vi "Sistema.vi"() -> ()   [LabVIEW 2017]
uses:
  <vilib>/Motion/Express/_s/nimc.ex.write.writeSetpoint.axis.vi
  <vilib>/Motion/Express/_s/nimc.fb.straightLineMove.startStraightLineMove.axis.modeAbsolute.0.vi
  <vilib>/Motion/Express/_s/nimc.ex.read.readExecutionData.axis.vi
  <vilib>/Motion/BlockNode/FB.NIMotion.xnode
panel:
  in  "Velocidad":dbl=10.0 format="%#_13g"
  out "x > y?":bool=TRUE
  out "done":bool=TRUE
  in  "Posición Inicial":cluster{"X":dbl, "Y":dbl, "Z":dbl}
  in  "Array":T1(array[cluster])=[{"Tipo Movimiento"=enum."Lineal", "X"=3.0, "Y"=0.0}, {"Tipo Movimiento"=enum."Lineal", "X"=3.0, "Y"=1.0}, {"Tipo Movimiento"=enum."Lineal", "X"=1.0, "Y"=1.0}, {"Tipo Movimiento"=enum."Lineal", "X"=1.0, "Y"=5.0}, {"Tipo Movimiento"=enum."Lineal", "X"=0.0, "Y"=5.0}, {"Tipo Movimiento"=enum."Lineal", "X"=0.0, "Y"=0.0}, {"Tipo Movimiento"=enum."Lineal", "X"=7.0, "Y"=0.0}, {"Tipo Movimiento"=enum."Lineal", "X"=7.0, "Y"=5.0}, {"Tipo Movimiento"=enum."Lineal", "X"=6.0, "Y"=5.0}, {"Tipo Movimiento"=enum."Lineal", "X"=6.0, "Y"=1.0}, {"Tipo Movimiento"=enum."Lineal", "X"=5.0, "Y"=1.0}, {"Tipo Movimiento"=enum."Lineal", "X"=5.0, "Y"=5.0}, {"Tipo Movimiento"=enum."Lineal", "X"=4.0, "Y"=5.0}, {"Tipo Movimiento"=enum."Lineal", "X"=4.0, "Y"=0.0}, {"Tipo Movimiento"=enum."Lineal", "X"=12.0, "Y"=0.0}, {"Tipo Movimiento"=enum."Lineal", "X"=12.0, "Y"=1.0}, {"Tipo Movimiento"=enum."Lineal", "X"=10.5, "Y"=1.0}, {"Tipo Movimiento"=enum."Lineal", "X"=10.5, "Y"=4.0}, {"Tipo Movimiento"=enum."Lineal", "X"=12.0, "Y"=4.0}, {"Tipo Movimiento"=enum."Lineal", "X"=12.0, "Y"=5.0}, {"Tipo Movimiento"=enum."Lineal", "X"=8.0, "Y"=5.0}, {"Tipo Movimiento"=enum."Lineal", "X"=8.0, "Y"=4.0}, {"Tipo Movimiento"=enum."Lineal", "X"=9.5, "Y"=4.0}, {"Tipo Movimiento"=enum."Lineal", "X"=9.5, "Y"=1.0}, {"Tipo Movimiento"=enum."Lineal", "X"=8.0, "Y"=1.0}, {"Tipo Movimiento"=enum."Lineal", "X"=8.0, "Y"=0.0}, {"Tipo Movimiento"=enum."Lineal", "X"=15.5, "Y"=0.0}, {"Tipo Movimiento"=enum."Lineal", "X"=16.0, "Y"=0.5}, {"Tipo Movimiento"=enum."Lineal", "X"=16.0, "Y"=2.0}, {"Tipo Movimiento"=enum."Lineal", "X"=15.5, "Y"=2.5}, {"Tipo Movimiento"=enum."Lineal", "X"=14.5, "Y"=2.5}, {"Tipo Movimiento"=enum."Lineal", "X"=14.0, "Y"=3.0}, {"Tipo Movimiento"=enum."Lineal", "X"=14.0, "Y"=3.5}, {"Tipo Movimiento"=enum."Lineal", "X"=14.5, "Y"=4.0}, {"Tipo Movimiento"=enum."Lineal", "X"=15.75, "Y"=4.0}, {"Tipo Movimiento"=enum."Lineal", "X"=16.0, "Y"=4.25}, {"Tipo Movimiento"=enum."Lineal", "X"=16.0, "Y"=4.75}, {"Tipo Movimiento"=enum."Lineal", "X"=15.75, "Y"=5.0}, {"Tipo Movimiento"=enum."Lineal", "X"=13.5, "Y"=5.0}, {"Tipo Movimiento"=enum."Lineal", "X"=13.0, "Y"=4.5}, {"Tipo Movimiento"=enum."Lineal", "X"=13.0, "Y"=2.5}, {"Tipo Movimiento"=enum."Lineal", "X"=13.5, "Y"=2.0}, {"Tipo Movimiento"=enum."Lineal", "X"=14.5, "Y"=2.0}, {"Tipo Movimiento"=enum."Lineal", "X"=15.0, "Y"=1.5}, {"Tipo Movimiento"=enum."Lineal", "X"=15.0, "Y"=1.0}, {"Tipo Movimiento"=enum."Lineal", "X"=14.5, "Y"=0.5}, {"Tipo Movimiento"=enum."Lineal", "X"=13.0, "Y"=0.5}, {"Tipo Movimiento"=enum."Lineal", "X"=13.0, "Y"=0.0}, {"Tipo Movimiento"=enum."Lineal", "X"=20.0, "Y"=0.0}, {"Tipo Movimiento"=enum."Lineal", "X"=20.0, "Y"=2.0}, {"Tipo Movimiento"=enum."Lineal", "X"=22.0, "Y"=2.0}, {"Tipo Movimiento"=enum."Lineal", "X"=22.0, "Y"=3.0}, {"Tipo Movimiento"=enum."Lineal", "X"=20.0, "Y"=3.0}, {"Tipo Movimiento"=enum."Lineal", "X"=20.0, "Y"=4.0}, {"Tipo Movimiento"=enum."Lineal", "X"=22.0, "Y"=4.0}, {"Tipo Movimiento"=enum."Lineal", "X"=22.0, "Y"=5.0}, {"Tipo Movimiento"=enum."Lineal", "X"=19.0, "Y"=5.0}, {"Tipo Movimiento"=enum."Lineal", "X"=19.0, "Y"=0.0}, {"Tipo Movimiento"=enum."Lineal", "X"=26.0, "Y"=0.0}, {"Tipo Movimiento"=enum."Lineal", "X"=26.0, "Y"=1.0}, {"Tipo Movimiento"=enum."Lineal", "X"=24.0, "Y"=1.0}, {"Tipo Movimiento"=enum."Lineal", "X"=24.0, "Y"=2.0}, {"Tipo Movimiento"=enum."Lineal", "X"=26.0, "Y"=2.0}, {"Tipo Movimiento"=enum."Lineal", "X"=26.0, "Y"=3.0}, {"Tipo Movimiento"=enum."Lineal", "X"=24.0, "Y"=3.0}, {"Tipo Movimiento"=enum."Lineal", "X"=24.0, "Y"=4.0}, {"Tipo Movimiento"=enum."Lineal", "X"=26.0, "Y"=4.0}, {"Tipo Movimiento"=enum."Lineal", "X"=26.0, "Y"=5.0}, {"Tipo Movimiento"=enum."Lineal", "X"=23.0, "Y"=5.0}, {"Tipo Movimiento"=enum."Lineal", "X"=23.0, "Y"=0.0}, {"Tipo Movimiento"=enum."Lineal", "X"=27.5, "Y"=0.0}, {"Tipo Movimiento"=enum."Lineal", "X"=27.5, "Y"=2.0}, {"Tipo Movimiento"=enum."Lineal", "X"=28.0, "Y"=2.0}, {"Tipo Movimiento"=enum."Lineal", "X"=29.0, "Y"=0.0}, {"Tipo Movimiento"=enum."Lineal", "X"=30.0, "Y"=0.0}, {"Tipo Movimiento"=enum."Lineal", "X"=30.0, "Y"=1.0}, {"Tipo Movimiento"=enum."Lineal", "X"=29.0, "Y"=2.5}]
  out "Paso":i32=69
  in  "Stop Button":bool
  out "EY":dbl(slide) scale=0.0..10.0
  out "EX":dbl(slide)=23.0 scale=0.0..10.0
  out "XY Graph":cluster{dbl[], dbl[]}(graph)={[0.0, 0.426423996, 1.426315789, 2.4263157890000002, 2.999891794, 3.0, 2.997709298, 2.215789474, 1.218080176, 1.0, 1.0, 1.0, 1.0, 1.0, 1.0, 0.45789473700000005, -0.0, -0.0, -0.0, -0.0, -0.0, -0.0, -0.0, 0.005048895, 0.32563547000000004, 1.194736842, 2.194736842, 2.894736842, 3.894736842, 4.894736842, 5.894736842, 6.727090094, 6.998255176, 7.0, 7.0, 7.0, 7.0, 7.0, 7.0, 7.0, 6.557894737, 6.0, 6.0, 6.0, 6.0, 6.0, 6.0, 5.557894737, 5.0, 5.0, 5.0, 5.0, 5.0, 5.0, 5.0, 4.157894737, 4.0, 4.0, 4.0, 4.0, 4.0, 4.0, 4.0, 4.048989208, 4.516094471, 5.436842105, 6.436842105, 7.436842105, 8.436842105, 9.436842105, 10.436842105, 11.387852897, 11.920747634, 12.0, 12.0, 11.916385042, 10.936842105, 10.5, 10.5, 10.5, 10.5, 10.5, 11.063157895, 11.979542936, 12.0, 12.0, 11.995418596, 11.529091619999999, 10.531578947, 9.531578947, 8.532151623, 8.002487327, 8.0, 8.0, 8.763157895, 9.5, 9.5, 9.5, 9.5, 9.5, 9.136842105, 8.066802093, 8.0, 8.0, 8.055501693, 8.564273623, 9.515789474, 10.515789474, 11.515789474, 12.515789474, 13.515789474, 14.514486319, 15.27534626, 15.499221793, 15.990506967, 16.0, 16.0, 15.584, 15.057894737, 14.5, 14.0, 14.116, 14.607617729, 15.601898554, 15.999811191, 16.0, 15.75, 15.105263158, 14.105263158, 13.5, 13.0, 13.0, 13.0, 13.0, 13.509032779, 14.486361958, 14.990506967, 15.0, 14.5, 13.836842105, 13.001629181, 13.0, 13.092082839, 13.707674496, 14.694736842, 15.694736842, 16.694736842, 17.694736842, 18.694736842, 19.602654003, 19.987062346000002, 20.0, 20.0, 20.0, 20.111486611, 21.084210526, 21.972723915, 22.0, 22.0, 21.415789474, 20.415789474, 20.0, 20.0, 20.111486611, 21.084210526, 21.972723915, 22.0, 22.0, 21.573576004, 20.573684211, 19.573684211, 19.0, 19.0, 19.0, 19.0, 19.0, 19.0, 19.0, 19.0, 19.167646748, 19.896481666, 20.894736842, 21.894736842, 22.894736842, 23.894736842, 24.994549846, 25.780379567, 25.999747518, 26.0, 26.0, 25.315789474, 24.218080176, 24.0, 24.0, 24.284282664, 25.284210526, 25.999927862, 26.0, 25.997709298, 25.215789474, 24.218080176, 24.0, 24.0, 24.284282664, 25.284210526, 25.999927862, 26.0, 25.99898191, 25.373684211, 24.373684211, 23.3747023, 23.0, 23.0, 23.0, 23.0, 23.0, 23.0, 23.0], [0.0, 0.0, 0.0, 0.0, 0.0, 0.5421052630000001, 1.0, 1.0, 1.0, 1.004581404, 1.568565328, 2.568421053, 3.568421053, 4.563839648, 4.999855725, 5.0, 5.0, 4.721283472, 3.789473684, 2.789473684, 1.6894736840000002, 0.689840197, 0.039900739000000005, 0.0, 0.0, 0.0, 0.0, 0.0, 0.0, 0.0, 0.0, 0.0, 0.0, 0.045163897, 0.71070666, 1.7105263160000002, 2.710526316, 3.610526316, 4.587072946, 4.997899781, 5.0, 5.0, 4.621142376, 3.631578947, 2.631578947, 1.532151623, 1.002487327, 1.0, 1.0, 1.3788576240000001, 2.268421053, 2.968421053, 3.868421053, 4.801204409, 5.0, 5.0, 4.97654663, 4.28929334, 3.289473684, 2.289473684, 1.289473684, 0.334637581, 0.000180344, 0.0, 0.0, 0.0, 0.0, 0.0, 0.0, 0.0, 0.0, 0.0, 0.0, 0.0, 0.742105263, 1.0, 1.0, 1.0, 1.5263157889999999, 2.526315789, 3.526315789, 4.0, 4.0, 4.0, 4.442105263, 5.0, 5.0, 5.0, 5.0, 5.0, 5.0, 5.0, 4.557894737, 4.0, 4.0, 4.0, 3.670425848, 2.6736842110000003, 1.673684211, 1.003258362, 1.0, 1.0, 0.657894737, -0.0, -0.0, -0.0, -0.0, -0.0, -0.0, -0.0, -0.0, -0.0, -0.0, -0.0, 0.490506967, 0.963157895, 1.933197907, 2.416, 2.5, 2.5, 3.025493033, 3.616, 4.0, 4.0, 4.249811191, 4.75, 5.0, 5.0, 5.0, 5.0, 4.5, 3.9157894740000003, 2.9157894740000003, 2.5, 2.0, 2.0, 1.509493033, 1.0, 0.5, 0.5, 0.5, 0.0, 0.0, 0.0, 0.0, 0.0, 0.0, 0.0, 0.0, 0.0, 0.0, 0.05435941800000001, 0.984210526, 1.929851108, 2.0, 2.0, 2.0, 2.342105263, 3.0, 3.0, 3.0, 3.0, 3.842105263, 4.0, 4.0, 4.0, 4.342105263, 5.0, 5.0, 5.0, 5.0, 5.0, 4.839704524, 3.989473684, 2.989473684, 1.989473684, 0.989473684, 0.14976916, -0.0, -0.0, -0.0, -0.0, -0.0, -0.0, -0.0, -0.0, -0.0, -0.0, 0.442105263, 1.0, 1.0, 1.0, 1.055743306, 1.986361958, 2.0, 2.0, 2.0, 2.542105263, 3.0, 3.0, 3.0, 3.055743306, 3.986361958, 4.0, 4.0, 4.0, 4.542105263, 5.0, 5.0, 5.0, 5.0, 5.0, 4.721283472, 3.789473684, 2.789473684, 1.789473684, 0.7894736840000001, 0.068190212]}
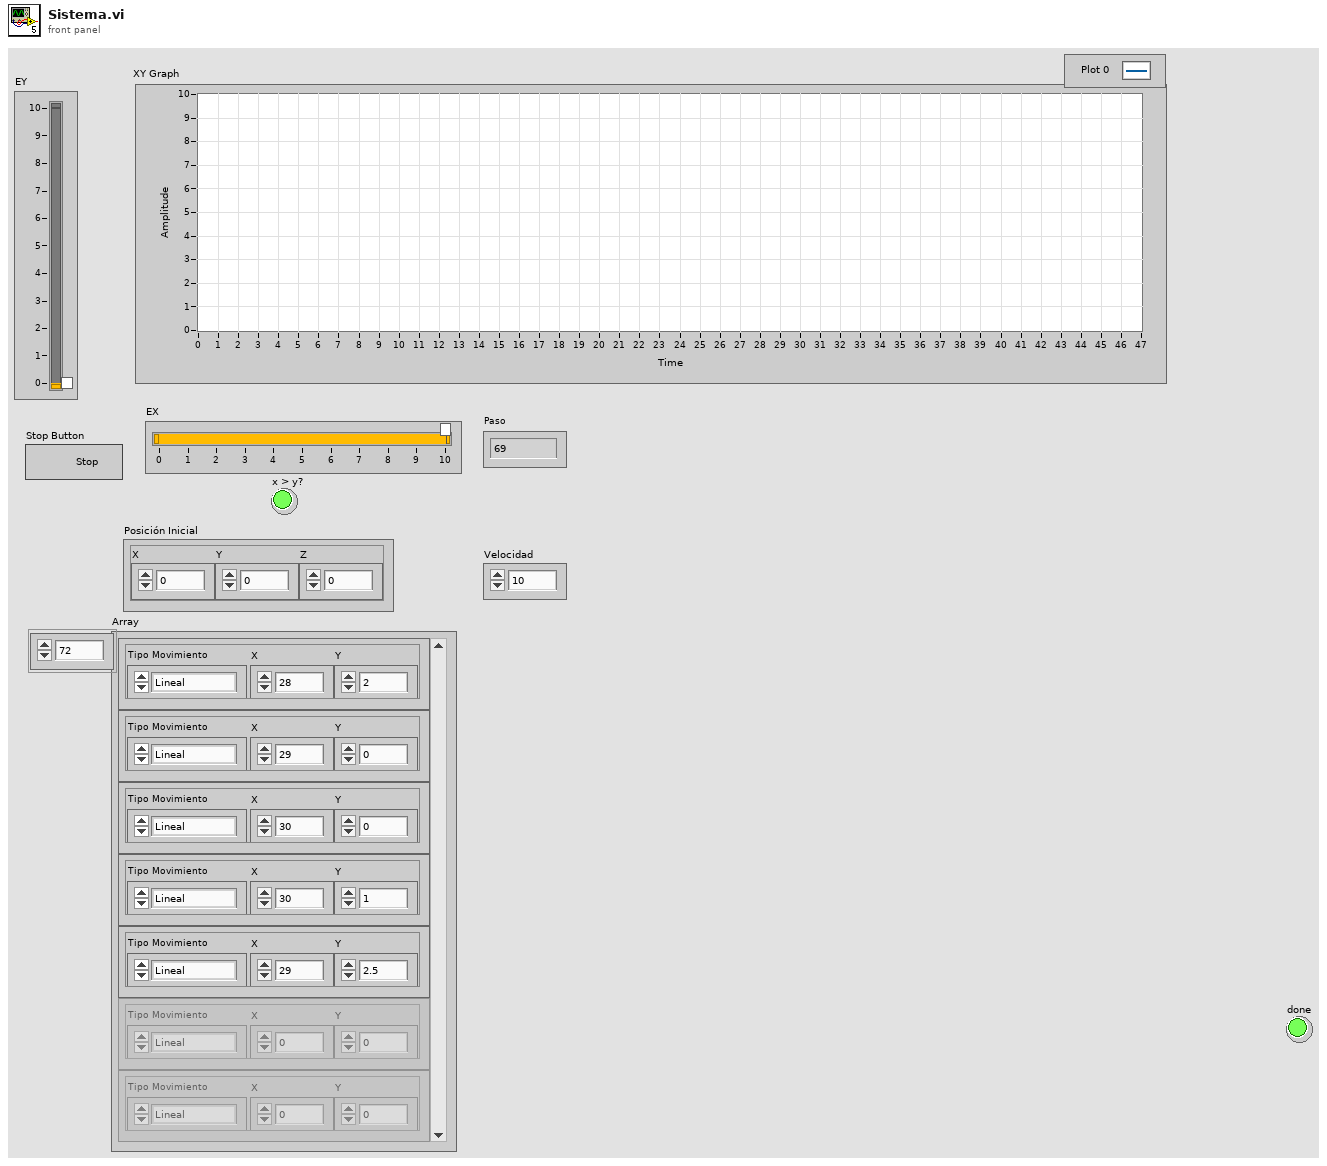
[diagram p1: front panel]
types:
  T1 = cluster{"Tipo Movimiento":enum16{"Lineal", "Circular"}, "X":dbl, "Y":dbl}[]
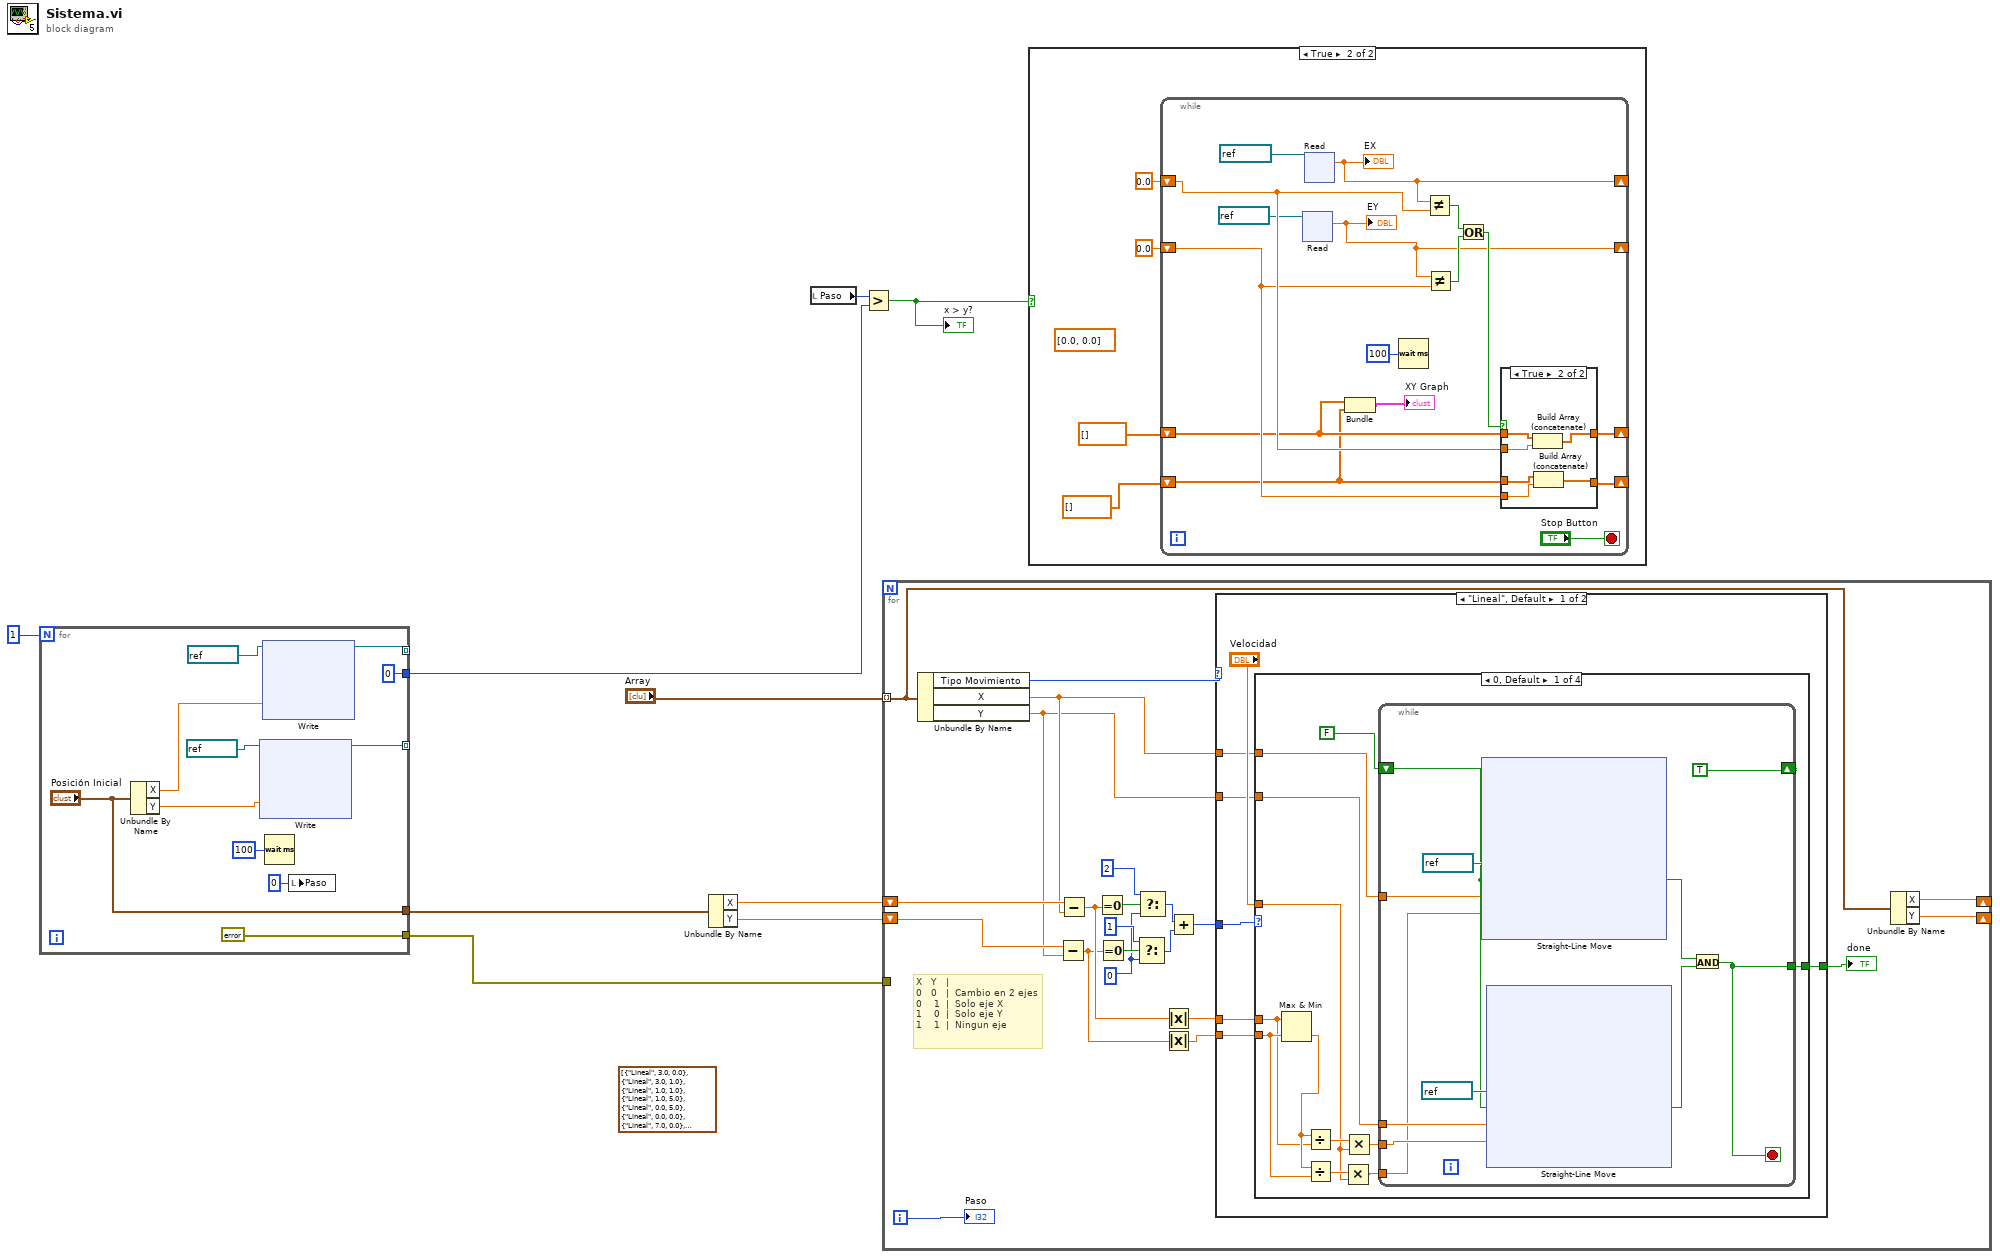
[diagram p0: block diagram]
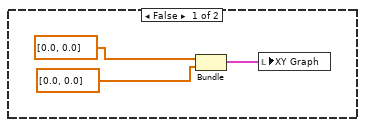
[diagram p2: hidden frame]
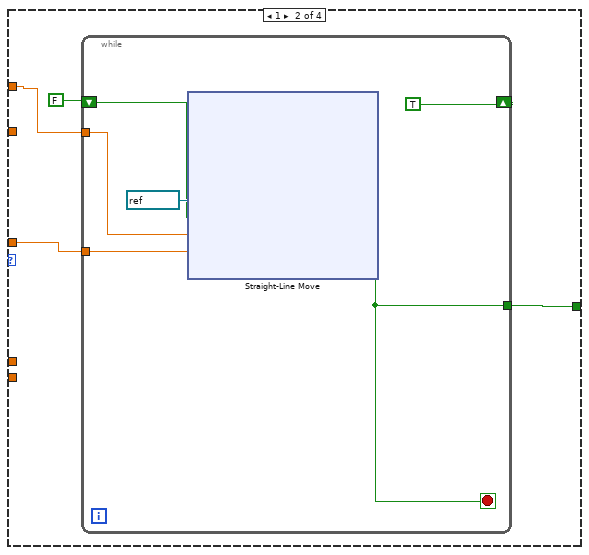
[diagram p4: hidden frame]
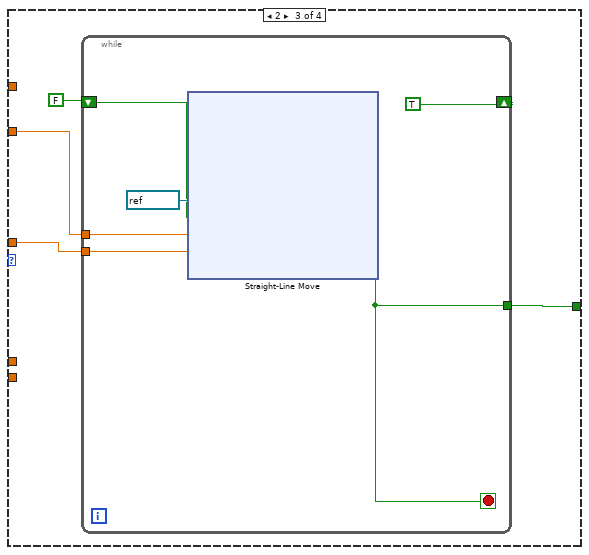
[diagram p5: hidden frame]
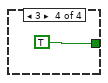
[diagram p6: hidden frame]
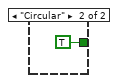
[diagram p7: hidden frame]
diagram:
  (unwired) T1 [{"Tipo Movimiento"=enum."Lineal", "X"=3.0, "Y"=0.0}, {"Tipo Movimiento"=enum."Lineal", "X"=3.0, "Y"=1.0}, {"Tipo Movimiento"=enum."Lineal", "X"=1.0, "Y"=1.0}, {"Tipo Movimiento"=enum."Lineal", "X"=1.0, "Y"=5.0}, {"Tipo Movimiento"=enum."Lineal", "X"=0.0, "Y"=5.0}, {"Tipo Movimiento"=enum."Lineal", "X"=0.0, "Y"=0.0}, {"Tipo Movimiento"=enum."Lineal", "X"=7.0, "Y"=0.0}, {"Tipo Movimiento"=enum."Lineal", "X"=7.0, "Y"=5.0}, {"Tipo Movimiento"=enum."Lineal", "X"=6.0, "Y"=5.0}, {"Tipo Movimiento"=enum."Lineal", "X"=6.0, "Y"=1.0}, {"Tipo Movimiento"=enum."Lineal", "X"=5.0, "Y"=1.0}, {"Tipo Movimiento"=enum."Lineal", "X"=5.0, "Y"=5.0}, {"Tipo Movimiento"=enum."Lineal", "X"=4.0, "Y"=5.0}, {"Tipo Movimiento"=enum."Lineal", "X"=4.0, "Y"=0.0}, {"Tipo Movimiento"=enum."Lineal", "X"=12.0, "Y"=0.0}, {"Tipo Movimiento"=enum."Lineal", "X"=12.0, "Y"=1.0}, {"Tipo Movimiento"=enum."Lineal", "X"=10.5, "Y"=1.0}, {"Tipo Movimiento"=enum."Lineal", "X"=10.5, "Y"=4.0}, {"Tipo Movimiento"=enum."Lineal", "X"=12.0, "Y"=4.0}, {"Tipo Movimiento"=enum."Lineal", "X"=12.0, "Y"=5.0}, {"Tipo Movimiento"=enum."Lineal", "X"=8.0, "Y"=5.0}, {"Tipo Movimiento"=enum."Lineal", "X"=8.0, "Y"=4.0}, {"Tipo Movimiento"=enum."Lineal", "X"=9.5, "Y"=4.0}, {"Tipo Movimiento"=enum."Lineal", "X"=9.5, "Y"=1.0}, {"Tipo Movimiento"=enum."Lineal", "X"=8.0, "Y"=1.0}, {"Tipo Movimiento"=enum."Lineal", "X"=8.0, "Y"=0.0}, {"Tipo Movimiento"=enum."Lineal", "X"=15.5, "Y"=0.0}, {"Tipo Movimiento"=enum."Lineal", "X"=16.0, "Y"=0.5}, {"Tipo Movimiento"=enum."Lineal", "X"=16.0, "Y"=2.0}, {"Tipo Movimiento"=enum."Lineal", "X"=15.5, "Y"=2.5}, {"Tipo Movimiento"=enum."Lineal", "X"=14.5, "Y"=2.5}, {"Tipo Movimiento"=enum."Lineal", "X"=14.0, "Y"=3.0}, {"Tipo Movimiento"=enum."Lineal", "X"=14.0, "Y"=3.5}, {"Tipo Movimiento"=enum."Lineal", "X"=14.5, "Y"=4.0}, {"Tipo Movimiento"=enum."Lineal", "X"=15.75, "Y"=4.0}, {"Tipo Movimiento"=enum."Lineal", "X"=16.0, "Y"=4.25}, {"Tipo Movimiento"=enum."Lineal", "X"=16.0, "Y"=4.75}, {"Tipo Movimiento"=enum."Lineal", "X"=15.75, "Y"=5.0}, {"Tipo Movimiento"=enum."Lineal", "X"=13.5, "Y"=5.0}, {"Tipo Movimiento"=enum."Lineal", "X"=13.0, "Y"=4.5}, {"Tipo Movimiento"=enum."Lineal", "X"=13.0, "Y"=2.5}, {"Tipo Movimiento"=enum."Lineal", "X"=13.5, "Y"=2.0}, {"Tipo Movimiento"=enum."Lineal", "X"=14.5, "Y"=2.0}, {"Tipo Movimiento"=enum."Lineal", "X"=15.0, "Y"=1.5}, {"Tipo Movimiento"=enum."Lineal", "X"=15.0, "Y"=1.0}, {"Tipo Movimiento"=enum."Lineal", "X"=14.5, "Y"=0.5}, {"Tipo Movimiento"=enum."Lineal", "X"=13.0, "Y"=0.5}, {"Tipo Movimiento"=enum."Lineal", "X"=13.0, "Y"=0.0}, {"Tipo Movimiento"=enum."Lineal", "X"=20.0, "Y"=0.0}, {"Tipo Movimiento"=enum."Lineal", "X"=20.0, "Y"=2.0}, {"Tipo Movimiento"=enum."Lineal", "X"=22.0, "Y"=2.0}, {"Tipo Movimiento"=enum."Lineal", "X"=22.0, "Y"=3.0}, {"Tipo Movimiento"=enum."Lineal", "X"=20.0, "Y"=3.0}, {"Tipo Movimiento"=enum."Lineal", "X"=20.0, "Y"=4.0}, {"Tipo Movimiento"=enum."Lineal", "X"=22.0, "Y"=4.0}, {"Tipo Movimiento"=enum."Lineal", "X"=22.0, "Y"=5.0}, {"Tipo Movimiento"=enum."Lineal", "X"=19.0, "Y"=5.0}, {"Tipo Movimiento"=enum."Lineal", "X"=19.0, "Y"=0.0}, {"Tipo Movimiento"=enum."Lineal", "X"=26.0, "Y"=0.0}, {"Tipo Movimiento"=enum."Lineal", "X"=26.0, "Y"=1.0}, {"Tipo Movimiento"=enum."Lineal", "X"=24.0, "Y"=1.0}, {"Tipo Movimiento"=enum."Lineal", "X"=24.0, "Y"=2.0}, {"Tipo Movimiento"=enum."Lineal", "X"=26.0, "Y"=2.0}, {"Tipo Movimiento"=enum."Lineal", "X"=26.0, "Y"=3.0}, {"Tipo Movimiento"=enum."Lineal", "X"=24.0, "Y"=3.0}, {"Tipo Movimiento"=enum."Lineal", "X"=24.0, "Y"=4.0}, {"Tipo Movimiento"=enum."Lineal", "X"=26.0, "Y"=4.0}, {"Tipo Movimiento"=enum."Lineal", "X"=26.0, "Y"=5.0}, {"Tipo Movimiento"=enum."Lineal", "X"=23.0, "Y"=5.0}, {"Tipo Movimiento"=enum."Lineal", "X"=23.0, "Y"=0.0}, {"Tipo Movimiento"=enum."Lineal", "X"=27.5, "Y"=0.0}, {"Tipo Movimiento"=enum."Lineal", "X"=27.5, "Y"=2.0}, {"Tipo Movimiento"=enum."Lineal", "X"=28.0, "Y"=2.0}, {"Tipo Movimiento"=enum."Lineal", "X"=29.0, "Y"=0.0}, {"Tipo Movimiento"=enum."Lineal", "X"=30.0, "Y"=0.0}, {"Tipo Movimiento"=enum."Lineal", "X"=30.0, "Y"=1.0}, {"Tipo Movimiento"=enum."Lineal", "X"=29.0, "Y"=2.5}] ("Array 2")
  n1 = for {
    N: 1 -> [_]
    tunnel: [errorcluster {"status"=FALSE, "code"=0, "source"=""} ("error in")] -> w1
    tunnel: ["Posición Inicial"] -> w7
    tunnel: [w16] -> _ mode=indexing
    tunnel: [w15] -> _ mode=indexing
    tunnel: [0 ("y")] -> w2
    n2 = Unbundle By Name("Posición Inicial") -> ("X"=w14:dbl, "Y"=w13:dbl)
    n3 = xnode ("Write")("position setpoint"=w13, "resource"=refnum<k21> "Eje Y" ("Motion Resource")) -> ("resource out"=w16:refnum<k21>)  [unwired: 1 in, 1 out]
    n4 = xnode ("Write")("position setpoint"=w14, "resource"=refnum<k21> "Eje X" ("Motion Resource")) -> ("resource out"=w15:refnum<k21>)  [unwired: 1 in, 1 out]
    n5 = Wait (ms)(milliseconds to wait=u32 100) -> ()  [unwired: 1 out]
    n6 = local write "Paso"(0 ("Paso")) -> ()
  }
  n7 = Unbundle By Name(w7) -> ("X"=w6:dbl, "Y"=w5:dbl)
  n8 = local read "Paso"() -> (w4:i32)
  n9 = Greater?(x=w4, y=w2) -> (0:w3:bool)
  "x > y?" <- w3
  n10 = for {
    tunnel: "Array" -> [w50] mode=indexing
    tunnel: w1 -> [_]
    shift-right: [w48] -> _
    shift-left: w5 -> [w45]
    shift-right: [w49] -> _
    shift-left: w6 -> [w47]
    i -> [w51]
    w39 = 0 ("f")
    # "X   Y   |\n0   0   |  Cambio en 2 ejes\n0    1  |  Solo eje X\n1    0  |  Solo eje Y\n1    1  |  Ningun eje"
    n11 = Unbundle By Name(w50) -> ("Tipo Movimiento"=w52:enum16{"Lineal", "Circular"}, "X"=w46:dbl, "Y"=w44:dbl)
    n12 = Subtract(x=w45, y=w44) -> (x-y=w32:dbl)
    n13 = Subtract(x=w47, y=w46) -> (x-y=w33:dbl)
    n14 = Equal To 0?(x=w33) -> (x = 0?=w43:bool)
    n15 = Equal To 0?(x=w32) -> (x = 0?=w41:bool)
    n16 = Select(t=1, s=w41, f=w39) -> (s? t:f=w37:i32)
    n17 = Select(t=2, s=w43, f=w39) -> (s? t:f=w38:i32)
    n18 = Absolute Value(x=w33) -> (abs(x)=w34:dbl)
    n19 = Absolute Value(x=w32) -> (abs(x)=w31:dbl)
    n20 = Add(x=w38, y=w37) -> (x+y=w36:i32)
    n21 = case shown="\"Lineal\", Default" w52 {
      tunnel: w46 -> [w56 _]
      tunnel: w44 -> [w55 _]
      tunnel: w36 -> [w59 _]
      tunnel: [w58 TRUE ("done")] -> w35
      tunnel: w31 -> [w54 _]
      tunnel: w34 -> [w53 _]
      frame "Lineal", Default {
        n22 = case shown="0, Default" w59 {
          tunnel: [w70 w119 w146 TRUE] -> w58
          tunnel: "Velocidad" -> [w63 w118 w145 _]
          tunnel: w56 -> [w69 w117 _ _]
          tunnel: w55 -> [w68 _ w144 _]
          tunnel: w54 -> [w61 _ _ _]
          tunnel: w53 -> [w60 _ _ _]
          frame 0, Default {
            n23 = Max & Min(x=w60, y=w61) -> (min(x,y)=w62:dbl)  [unwired: 1 out]
            n24 = Divide(x=w62, y=w60) -> (x/y=w65:dbl)
            n25 = Divide(x=w62, y=w61) -> (x/y=w64:dbl)
            n26 = Multiply(x=w64, y=w63) -> (x*y=w67:dbl)
            n27 = Multiply(x=w65, y=w63) -> (x*y=w66:dbl)
            n28 = while {
              shift-right: [TRUE] -> _
              shift-left: FALSE -> [w79]
              tunnel: [w76] -> w70
              tunnel: w69 -> [w75]
              tunnel: w68 -> [w74]
              tunnel: w67 -> [w72]
              tunnel: w66 -> [w73]
              stop <- w76 stop-if-true
              n29 = xnode "Straight-Line Move"("resource"=refnum<k21> "Eje X" ("Motion Resource"), "execute"=w79, "position"=w75, "velocity"=w72) -> ("done"=w78:bool)  [unwired: 2 in, 2 out]
              n30 = xnode "Straight-Line Move"("resource"=refnum<k21> "Eje Y" ("Motion Resource"), "execute"=w79, "position"=w74, "velocity"=w73) -> ("done"=w77:bool)  [unwired: 2 in, 2 out]
              n31 = And(x=w78, y=w77) -> (x .and. y?=w76:bool)
            }
          }
          frame 1 {
            n32 = while {
              shift-right: [TRUE] -> _
              shift-left: FALSE -> [w124]
              tunnel: [w123] -> w119
              tunnel: w118 -> [w122]
              tunnel: w117 -> [w121]
              stop <- w123 stop-if-true
              n33 = xnode "Straight-Line Move"("resource"=refnum<k21> "Eje X" ("Motion Resource"), "execute"=w124, "position"=w121, "velocity"=w122) -> ("done"=w123:bool)  [unwired: 2 in, 2 out]
            }
          }
          frame 2 {
            n34 = while {
              shift-right: [TRUE] -> _
              shift-left: FALSE -> [w151]
              tunnel: [w150] -> w146
              tunnel: w145 -> [w149]
              tunnel: w144 -> [w148]
              stop <- w150 stop-if-true
              n35 = xnode "Straight-Line Move"("resource"=refnum<k21> "Eje Y" ("Motion Resource"), "execute"=w151, "position"=w148, "velocity"=w149) -> ("done"=w150:bool)  [unwired: 2 in, 2 out]
            }
          }
          frame 3 {
          }
        }
      }
      frame "Circular" {
      }
    }
    "done" <- w35
    n36 = Unbundle By Name(w50) -> ("X"=w49:dbl, "Y"=w48:dbl)
    "Paso" <- w51
  }
  n37 = case shown="True" w3 {
    frame False {
      n38 = Bundle(dbl[] [0.0, 0.0], dbl[] [0.0, 0.0]) -> (w173:cluster{dbl[], dbl[]})  [unwired: 1 in]
      n39 = local write "XY Graph"(w173) -> ()
    }
    frame True {
      (unwired) dbl[] [0.0, 0.0]
      n40 = while {
        shift-right: [w186] -> _
        shift-left: 0.0 ("position") -> [w192]
        shift-right: [w187] -> _
        shift-left: 0.0 ("position") -> [w191]
        shift-right: [w190] -> _
        shift-left: dbl[] [] -> [w183]
        shift-right: [w189] -> _
        shift-left: dbl[] [] -> [w184]
        stop <- "Stop Button" stop-if-true
        n41 = xnode "Read"("resource"=refnum<k21> "Eje Y" ("Motion Resource")) -> ("position"=w187:dbl)  [unwired: 1 in, 6 out]
        "EY" <- w187
        n42 = xnode "Read"("resource"=refnum<k21> "Eje X" ("Motion Resource")) -> ("position"=w186:dbl)  [unwired: 1 in, 6 out]
        "EX" <- w186
        n43 = Bundle(w184, w183) -> (→"XY Graph":cluster{dbl[], dbl[]})  [unwired: 1 in]
        n44 = Wait (ms)(milliseconds to wait=u32 100) -> ()  [unwired: 1 out]
        n45 = Not Equal?(x=w186, y=w192) -> (x != y?=w195:bool)
        n46 = Not Equal?(x=w187, y=w191) -> (x != y?=w194:bool)
        n47 = Or(x=w195, y=w194) -> (x .or. y?=w193:bool)
        n48 = case shown="True" w193 {
          tunnel: w184 -> [w197 w203]
          tunnel: w183 -> [w196 w200]
          tunnel: w192 -> [_ w202]
          tunnel: w191 -> [_ w199]
          tunnel: [w196 w198] -> w190
          tunnel: [w197 w201] -> w189
          frame False {
          }
          frame True {
            n49 = Build Array (concatenate)(w203, w202) -> (w201:dbl[])
            n50 = Build Array (concatenate)(w200, w199) -> (w198:dbl[])
          }
        }
      }
    }
  }
